vi "Two Axis Display.vi"(0 "Data In":T4 {"time" format="%<%.3X>T"}, 2 "Display State In":T2 {"Time_data" format="%<%.3X>T"}, 3 "Container State":T3) -> (6 "Data Out":T4 {"time" format="%<%.3X>T"}, 7 "Display State Out":T2 {"Time_data" format="%<%.3X>T"}, 8 "Action":T1)   [LabVIEW 2015, in "Two Axis.xctl"]
uses:
  Two Axis.xctl
  Two Axis Data.ctl
  <vilib>/_xctls/Container State.ctl
  Two Axis State.ctl
  <vilib>/_xctls/Action.ctl
  <vilib>/_xctls/XControlSupport.lvlib
panel:
  out "2_axis_Data":cluster{"Time_data":timestamp[], sgl[]}[](graph) caption="Vaisala Data"
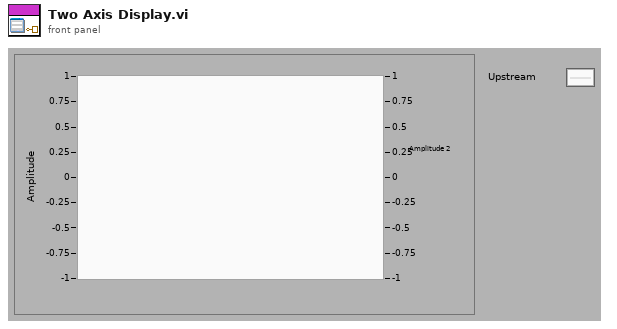
[diagram p1: front panel]
types:
  T1 = typedef "XControlSupport.lvlib/Action.ctl" = cluster{"Data Changed?":bool, "State Changed?":bool, "Action Name":string}
  T2 = typedef "Two Axis.xctl/Two Axis State.ctl" = cluster{"History":i32, "Time_data":timestamp[], "Data_Out":sgl[][], "NumPlots":i32, "LegElem":i32, "Plot Details":cluster{"Name":string, "Line Width":u8, "Line Style":u8, "Color":u32}[], "Y-Axis Labels":string[], "Title":string, "data_only?":bool}
  T3 = typedef "XControlSupport.lvlib/Container State.ctl" = cluster{"Indicator?":bool, "Run Mode?":bool, " Refnum":refnum<vi>}
  T4 = typedef "Two Axis.xctl/Two Axis Data.ctl" = cluster{"Data":sgl[], "time":timestamp}
  T5 = cluster{"Name":string, "Line Width":u8, "Line Style":u8, "Color":u32}[]
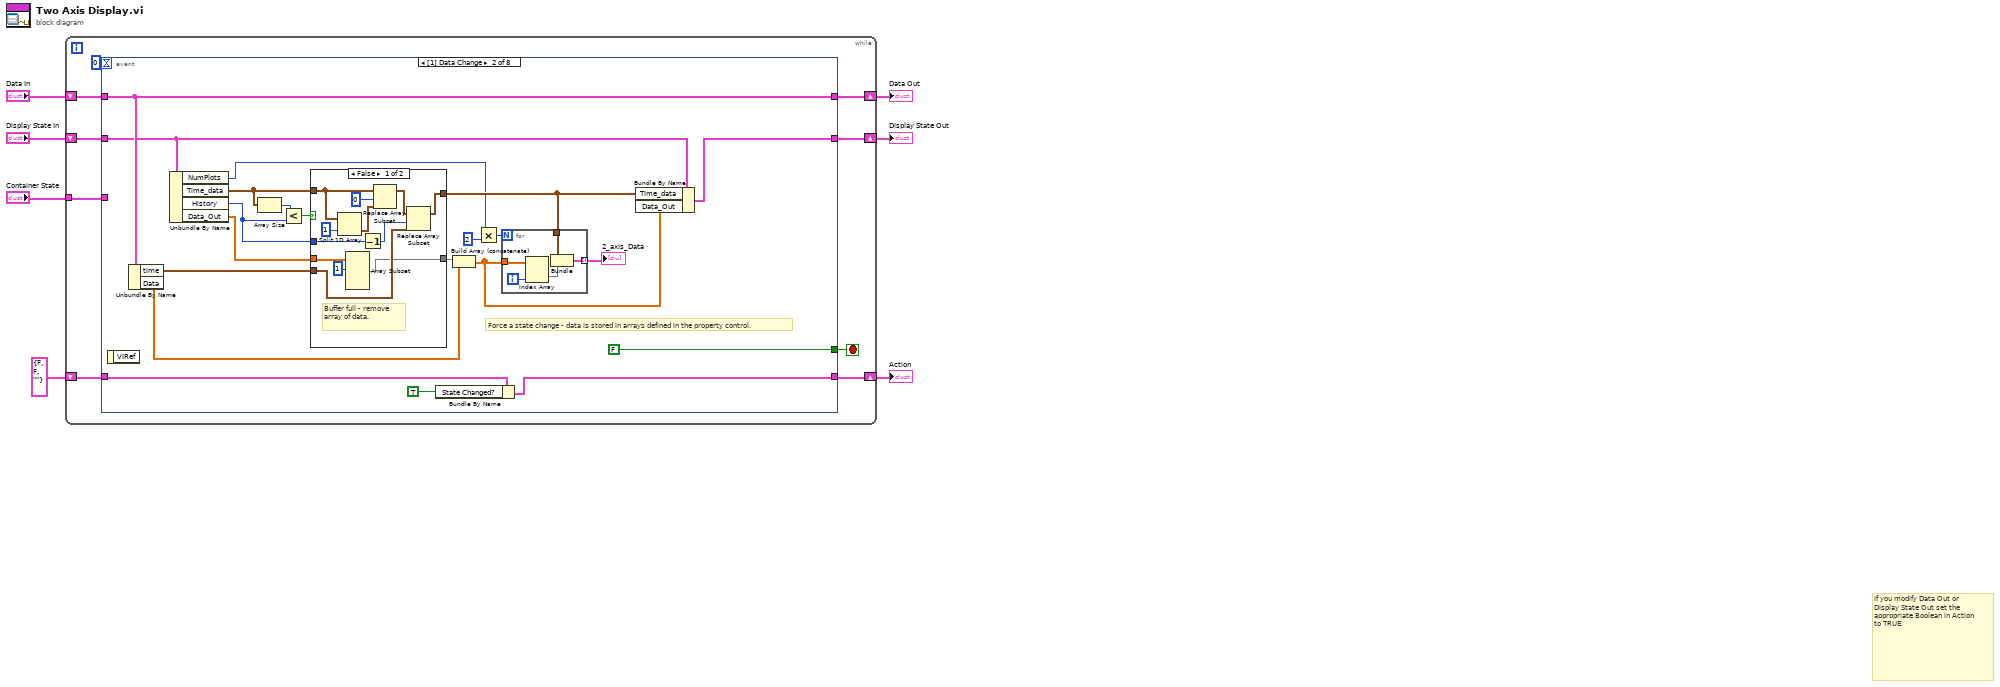
[diagram p0: block diagram]
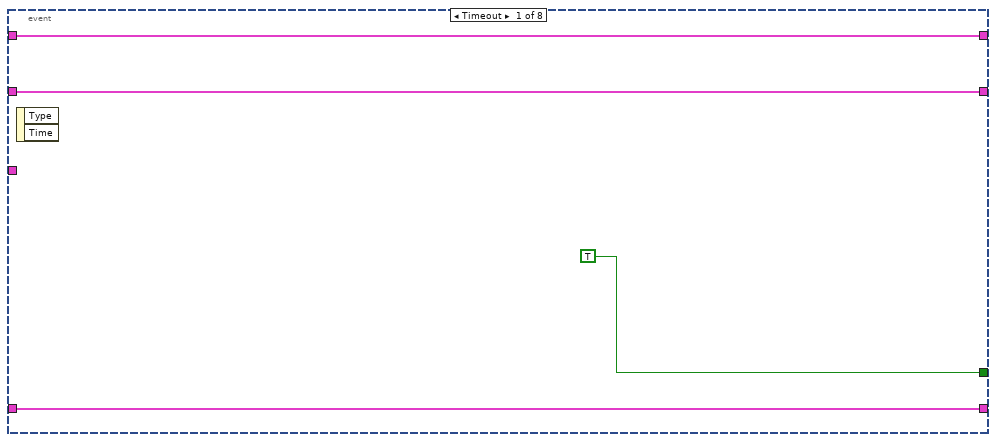
[diagram p2: hidden frame]
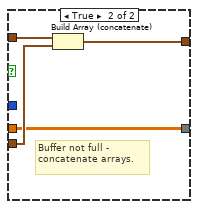
[diagram p3: hidden frame]
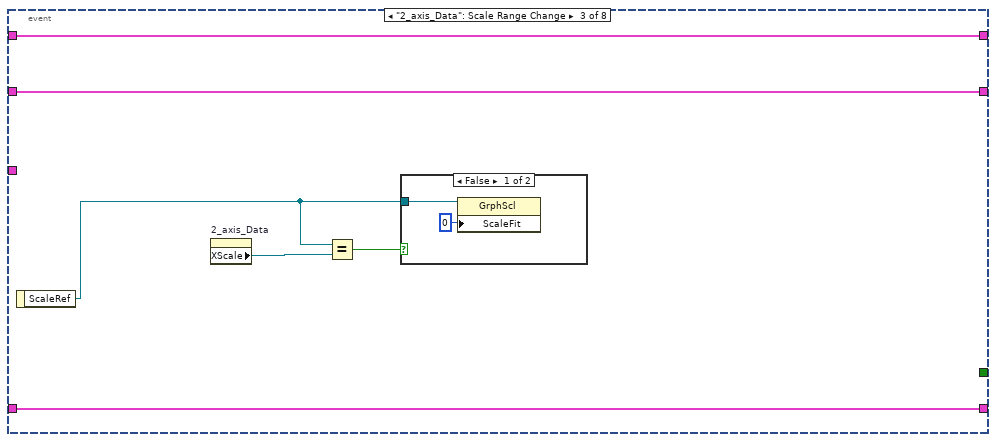
[diagram p4: hidden frame]
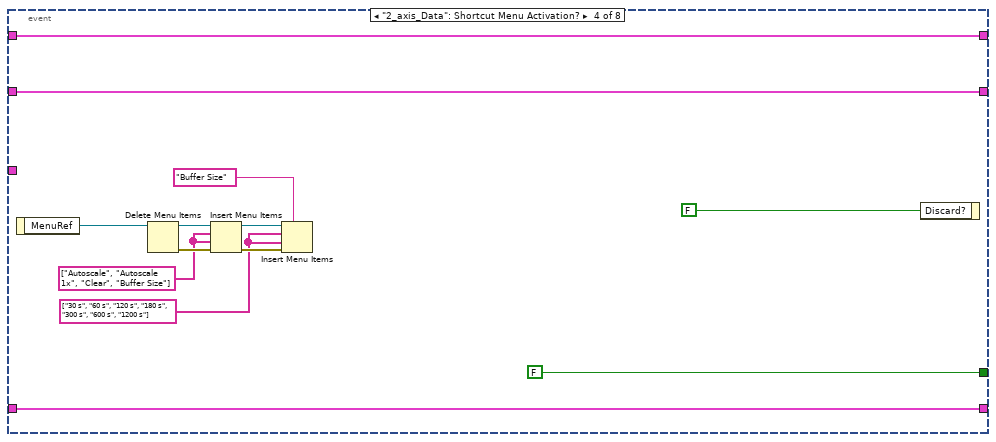
[diagram p6: hidden frame]
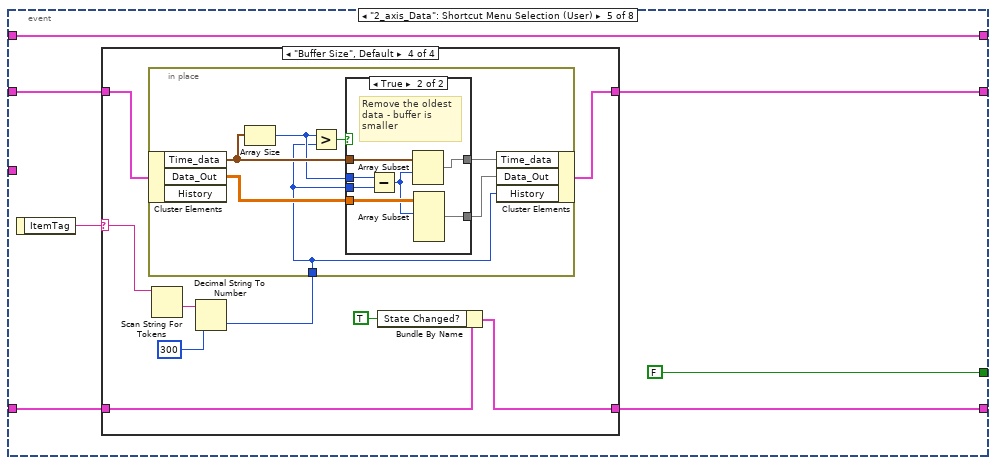
[diagram p7: hidden frame]
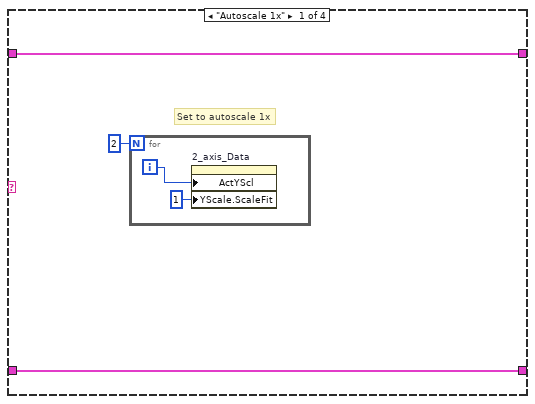
[diagram p8: hidden frame]
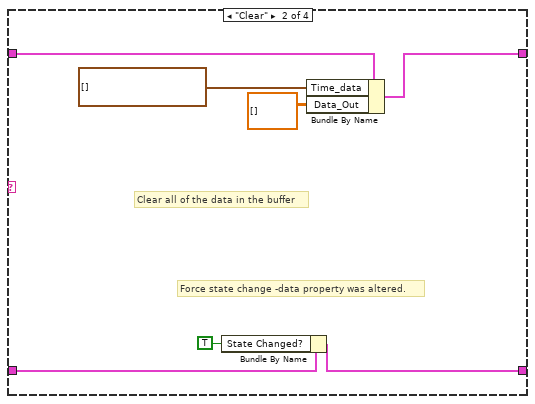
[diagram p9: hidden frame]
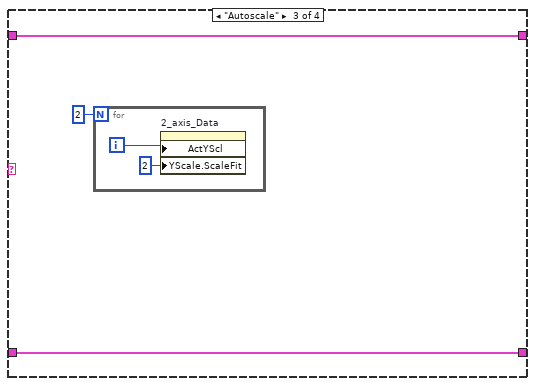
[diagram p10: hidden frame]
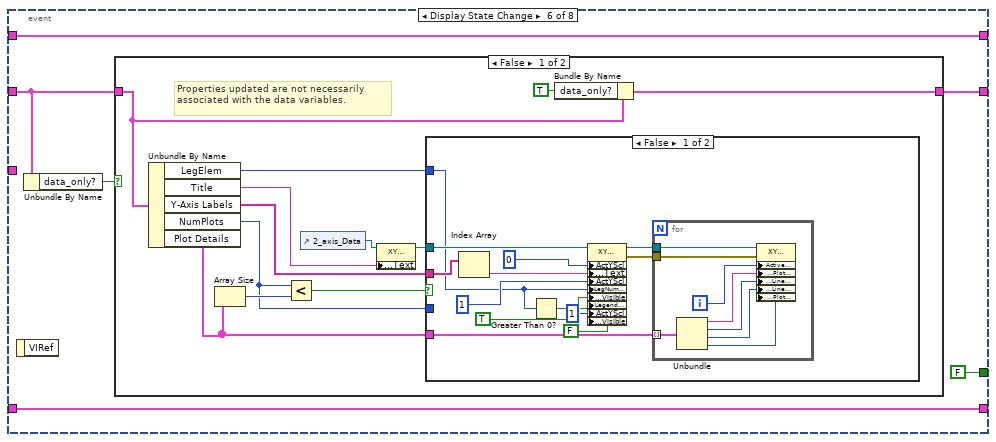
[diagram p12: hidden frame]
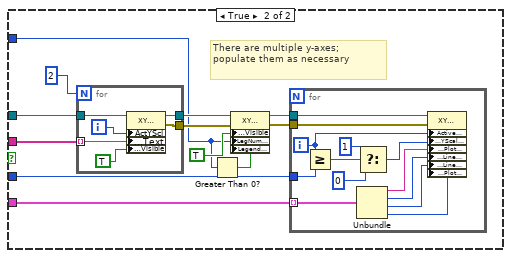
[diagram p13: hidden frame]
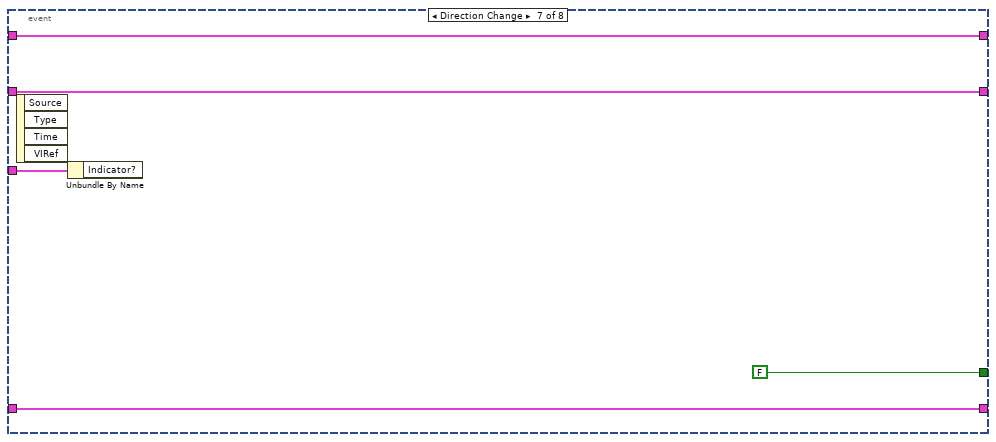
[diagram p15: hidden frame]
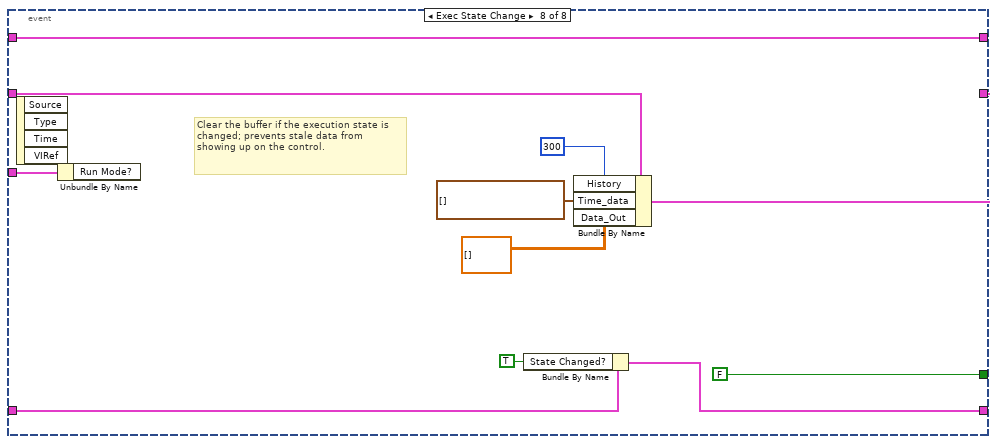
[diagram p16: hidden frame]
diagram:
  # "If you modify Data Out or\nDisplay State Out set the\nappropriate Boolean in Action\nto TRUE."
  n1 = while {
    shift-right: [w15] -> w4
    shift-left: "Display State In" -> [w16]
    tunnel: "Container State" -> [w12]
    shift-right: [w10] -> w7
    shift-left: "Data In" -> [w11]
    shift-right: [w8] -> w2
    shift-left: T1 {"Data Changed?"=FALSE, "State Changed?"=FALSE, "Action Name"=""} ("Action") -> [w9]
    stop <- w14 stop-if-true
    n2 = event shown="[1] Data Change" {
      selector: _ -> [_ _ _ _ _ _ _ _]
      dyn-events: _ -> [_ _ _ _ _ _ _ _]
      timeout: 0 -> [_ _ _ _ _ _ _ _]
      tunnel: w16 -> [w18 w31 w67 w83 w88 w135 w207 w217]
      tunnel: [w18 w28 w67 w83 w86 w134 w207 w210] -> w15
      tunnel: [TRUE FALSE _ FALSE FALSE FALSE FALSE FALSE] -> w14
      tunnel: w12 -> [_ _ _ _ _ _ w208 w219]
      tunnel: w11 -> [w17 w41 w68 w82 w90 w138 w206 w218]
      tunnel: [w17 w41 w68 w82 w90 w138 w206 w218] -> w10
      tunnel: [w19 w25 w66 w81 w85 w137 w205 w211] -> w8
      tunnel: w9 -> [w19 w27 w66 w81 w87 w137 w205 w213]
      event Timeout {
        n3 = event-data() -> ()  [unwired: 1 in, 2 out]
      }
      event Data Change {
        # "Force a state change - data is stored in arrays defined in the property control."
        n4 = event-data() -> ()  [unwired: 1 in, 1 out]
        n5 = Unbundle By Name(w41) -> ("time"=w40:timestamp, "Data"=w37:sgl[])
        n6 = Unbundle By Name(w31) -> ("NumPlots"=w23:i32, "Time_data"=w36:timestamp[], "History"=w34:i32, "Data_Out"=w38:sgl[][])
        n7 = Array Size(array=w36) -> (size(s)=w35:i32)
        n8 = Less?(x=w35, y=w34) -> (x < y?=w33:bool)
        n9 = case shown="False" w33 {
          tunnel: w36 -> [w53 w62]
          tunnel: [w52 w60] -> w30
          tunnel: w40 -> [w51 w61]
          tunnel: w38 -> [w48 w59]
          tunnel: w34 -> [w50 _]
          tunnel: [w47 w59] -> w39
          frame False {
            # "Buffer full - remove array of data."
            n10 = Split 1D Array(array=w53, index=1) -> (second subarray=w54:timestamp[])  [unwired: 1 out]
            n11 = Array Subset(array=w48, index (row)=1 ("index")) -> (w47:sgl[][])  [unwired: 3 in]
            n12 = Decrement(x=w50) -> (x-1=w56:i32)
            n13 = Replace Array Subset(array=w53, new element=w54, index=0) -> (w57:timestamp[])
            n14 = Replace Array Subset(array=w57, new element=w51, index=w56) -> (w52:timestamp[])
          }
          frame True {
            # "Buffer not full - concatenate arrays."
            n15 = Build Array (concatenate)(w62, w61) -> (w60:timestamp[])
          }
        }
        n16 = Bundle By Name(cluster=w27, "State Changed?"=TRUE) -> (w25:T1)
        n17 = Build Array (concatenate)(w39, w37) -> (w29:sgl[][])
        n18 = Multiply(x=w23, y=2) -> (x*y=w21:i32)
        n19 = for {
          N: w21 -> [_]
          tunnel: w29 -> [w46]
          tunnel: w30 -> [w44]
          tunnel: [w42] -> w32 mode=indexing
          i -> [w45]
          n20 = Index Array(array=w46, index (col)=w45) -> (element=w43:sgl[])  [unwired: 1 in]
          n21 = Bundle("Time_data"=w44, w43) -> (w42:cluster{"Time_data":timestamp[], sgl[]})  [unwired: 1 in]
        }
        "2_axis_Data" <- w32
        n22 = Bundle By Name(cluster=w31, "Time_data"=w30, "Data_Out"=w29) -> (w28:T2)
      }
      event "2_axis_Data": Scale Range Change {
        n23 = event-data() -> ("ScaleRef"=w64:refnum<vi>)  [unwired: 1 in]
        n24 = property on="2_axis_Data" class="XYGraph (strict)"() -> ("XScale"=w65:refnum<vi>)  [unwired: 2 in, 2 out]
        n25 = Equal?(x=w64, y=w65) -> (x = y?=w63:bool)
        n26 = case shown="False" w63 {
          tunnel: w64 -> [w69 _]
          frame False {
            n27 = property class="GrphScl"(reference=w69, "ScaleFit"=u8 0 ("Scale Fit")) -> ()  [unwired: 1 in, 2 out]
          }
          frame True {
          }
        }
      }
      event "2_axis_Data": Shortcut Menu Activation? {
        w71 = string[] ["Autoscale", "Autoscale 1x", "Clear", "Buffer Size"] ("item names")
        w72 = string[] ["30 s", "60 s", "120 s", "180 s", "300 s", "600 s", "1200 s"]
        n28 = event-data() -> ("MenuRef"=w78:refnum<k9>)  [unwired: 1 in]
        n29 = Delete Menu Items(9:w78) -> (0:w76:errorcluster, 3:w77:refnum<k9>)  [unwired: 3 in]
        n30 = Insert Menu Items(6:w76, 7:w71, 8:w71, 9:w77) -> (0:w74:errorcluster, 3:w75:refnum<k9>)  [unwired: 2 in, 1 out]
        n31 = Insert Menu Items(5:"Buffer Size", 6:w74, 7:w72, 8:w72, 9:w75) -> ()  [unwired: 1 in, 3 out]
        n32 = event-data("Discard?"=FALSE) -> ()  [unwired: 1 in, 1 out]
      }
      event "2_axis_Data": Shortcut Menu Selection (User) {
        n33 = event-data() -> ("ItemTag"=w89:string)  [unwired: 1 in]
        n34 = case shown="\"Buffer Size\", Default" w89 {
          selector: w89 -> [_ _ _ w114]
          tunnel: w88 -> [w93 w102 w105 w116]
          tunnel: w87 -> [w92 w98 w104 w110]
          tunnel: [w93 w99 w105 w115] -> w86
          tunnel: [w92 w97 w104 w108] -> w85
          frame "Autoscale 1x" {
            # "Set to autoscale 1x"
            n35 = for {
              N: 2 -> [_]
              i -> [w94]
              n36 = property on="2_axis_Data" class="XYGraph (strict)"("ActYScl"=w94, "YScale.ScaleFit"=u8 1 ("Y Scale.Scale Fit")) -> ()  [unwired: 2 in, 2 out]
            }
          }
          frame "Clear" {
            # "Force state change -data property was altered."
            # "Clear all of the data in the buffer"
            n37 = Bundle By Name(cluster=w98, "State Changed?"=TRUE) -> (w97:T1)
            n38 = Bundle By Name(cluster=w102, "Time_data"=timestamp[] [], "Data_Out"=sgl[][] []) -> (w99:T2)
          }
          frame "Autoscale" {
            n39 = for {
              N: 2 -> [_]
              i -> [w106]
              n40 = property on="2_axis_Data" class="XYGraph (strict)"("ActYScl"=w106, "YScale.ScaleFit"=u8 2 ("Y Scale.Scale Fit")) -> ()  [unwired: 2 in, 2 out]
            }
          }
          frame "Buffer Size", Default {
            n41 = Scan String For Tokens(9:w114) -> (1:w113:string)  [unwired: 5 in, 3 out]
            n42 = Decimal String To Number(string=w113, default (0L)=300 ("default (0 I32)")) -> (number=w111:i32)  [unwired: 1 in, 1 out]
            n43 = in-place {
              in-place-border: w111 -> [w117]
              n44 = in-place-cluster #1(w116) -> ("Time_data"=w122:timestamp[], "Data_Out"=w120:sgl[][])  [unwired: 1 out]
              n45 = Array Size(array=w122) -> (size(s)=w118:i32)
              n46 = Greater?(x=w118, y=w117) -> (0:w123:bool)
              n47 = case shown="True" w123 {
                tunnel: w122 -> [w125 w132]
                tunnel: [w125 w129] -> w121
                tunnel: w120 -> [w124 w128]
                tunnel: [w124 w127] -> w119
                tunnel: w118 -> [_ w131]
                tunnel: w117 -> [_ w130]
                frame False {
                  # "Buffer not filled yet or was smaller"
                }
                frame True {
                  # "Remove the oldest data - buffer is smaller"
                  n48 = Subtract(x=w131, y=w130) -> (x-y=w126:i32)
                  n49 = Array Subset(array=w132, index=w126) -> (w129:timestamp[])  [unwired: 1 in]
                  n50 = Array Subset(array=w128, index (row)=w126) -> (w127:sgl[][])  [unwired: 3 in]
                }
              }
              n51 = in-place-cluster #1("Time_data"=w121, "Data_Out"=w119, "History"=w117) -> (w115:T2)
            }
            n52 = Bundle By Name(cluster=w110, "State Changed?"=TRUE) -> (w108:T1)
          }
        }
      }
      event Display State Change {
        n53 = event-data() -> ()  [unwired: 1 in, 1 out]
        n54 = Unbundle By Name(w135) -> ("data_only?"=w136:bool)
        n55 = case shown="False" w136 {
          tunnel: w135 -> [w145 w203]
          tunnel: [w143 w203] -> w134
          frame False {
            # "Properties updated are not necessarily associated with the data variables."
            n56 = Unbundle By Name(w145) -> ("LegElem"=w146:i32, "Title"=w150:string, "Y-Axis Labels"=w139:string[], "NumPlots"=w141:i32, "Plot Details"=w140:T5)
            n57 = Array Size(array=w140) -> (size(s)=w142:i32)
            n58 = Less?(x=w141, y=w142) -> (x < y?=w148:bool)
            n59 = control-ref of="2_axis_Data"() -> (w149:refnum<vi>)
            n60 = property on="Property Node" class="XYGraph (strict)"(reference=w149, "Caption.Text"=w150) -> (reference out=w147:refnum<vi>)  [unwired: 1 in, 1 out]
            n61 = case shown="False" w148 {
              tunnel: w147 -> [w157 w182]
              tunnel: w139 -> [w162 w181]
              tunnel: w140 -> [w158 w177]
              tunnel: w141 -> [_ w176]
              tunnel: w146 -> [w154 w173]
              frame False {
                n62 = Index Array(array=w162) -> (element=w161:string)  [unwired: 1 in]
                n63 = Greater Than 0?(x=w154) -> (x > 0?=w153:bool)
                n64 = property class="XYGraph (strict)"(reference=w157, "ActYScl"=0 ("Active Y Scale"), "YScale.NameLbl.Text"=w161, "ActYScl"=1 ("Active Y Scale"), "LegNumRows"=w154, "YScale.Visible"=TRUE ("Y Scale.Visible"), "Legend Visible"=w153, "ActYScl"=1 ("Active Y Scale"), "YScale.Visible"=FALSE ("Y Scale.Visible")) -> (reference out=w159:refnum<vi>, error out=w155:errorcluster)  [unwired: 1 in]
                n65 = for {
                  tunnel: w159 -> [w171]
                  tunnel: w158 -> [w170] mode=indexing
                  tunnel: w155 -> [w164]
                  i -> [w168]
                  n66 = Unbundle(w170) -> ("Name"=w169:string, "Line Width"=w167:u8, "Line Style"=w166:u8, "Color"=w165:u32)
                  n67 = property class="XYGraph (strict)"(reference=w171, error in=w164, "Active Plot"=w168, "Plot.Plot Name"=w169, "Plot.Line Width"=w167, "Plot.Line Style"=w166, "Plot.Plot Color"=w165) -> ()  [unwired: 2 out]
                }
              }
              frame True {
                # "There are multiple y-axes; populate them as necessary"
                n68 = for {
                  N: 2 -> [_]
                  tunnel: w182 -> [w202]
                  tunnel: w181 -> [w200] mode=indexing
                  tunnel: [w199] -> w180
                  tunnel: [w197] -> w174
                  i -> [w201]
                  n69 = property class="XYGraph (strict)"(reference=w202, "ActYScl"=w201, "YScale.NameLbl.Text"=w200, "YScale.Visible"=TRUE ("Y Scale.Visible")) -> (reference out=w199:refnum<vi>, error out=w197:errorcluster)  [unwired: 1 in]
                }
                n70 = Greater Than 0?(x=w173) -> (x > 0?=w172:bool)
                n71 = property class="XYGraph (strict)"(reference=w180, error in=w174, "YScale.Visible"=TRUE ("Y Scale.Visible"), "LegNumRows"=w173, "Legend Visible"=w172) -> (reference out=w178:refnum<vi>, error out=w175:errorcluster)
                n72 = for {
                  tunnel: w178 -> [w196]
                  tunnel: w177 -> [w189] mode=indexing
                  tunnel: w176 -> [w194]
                  tunnel: w175 -> [w184]
                  i -> [w195]
                  n73 = Greater Or Equal?(x=w195, y=w194) -> (x >= y?=w193:bool)
                  n74 = Unbundle(w189) -> ("Name"=w188:string, "Line Width"=w187:u8, "Line Style"=w186:u8, "Color"=w185:u32)
                  n75 = Select(t=u32 1, s=w193, f=u32 0 ("Plot.Y Scale Index")) -> (s? t:f=w190:u32)
                  n76 = property class="XYGraph (strict)"(reference=w196, error in=w184, "Active Plot"=w195, "Plot.YScaleIdx"=w190, "Plot.Plot Name"=w188, "Plot.Line Width"=w187, "Plot.Line Style"=w186, "Plot.Plot Color"=w185) -> ()  [unwired: 2 out]
                }
              }
            }
            n77 = Bundle By Name(cluster=w145, "data_only?"=TRUE) -> (w143:T2)
          }
          frame True {
          }
        }
      }
      event Direction Change {
        n78 = event-data() -> ()  [unwired: 1 in, 4 out]
        n79 = Unbundle By Name(w208) -> ()  [unwired: 1 out]
      }
      event Exec State Change {
        # "Clear the buffer if the execution state is changed; prevents stale data from showing up on the control."
        n80 = event-data() -> ()  [unwired: 1 in, 4 out]
        n81 = Unbundle By Name(w219) -> ()  [unwired: 1 out]
        n82 = Bundle By Name(cluster=w213, "State Changed?"=TRUE) -> (w211:T1)
        n83 = Bundle By Name(cluster=w217, "History"=300, "Time_data"=timestamp[] [], "Data_Out"=sgl[][] []) -> (w210:T2)
      }
    }
  }
  "Display State Out" <- w4
  "Data Out" <- w7
  "Action" <- w2
